vi "Actor Core.vi"(8 "error in":errorcluster, 11 "CANopen Test UI in":refnum<class "CANopen Test UI Actor.lvclass">) -> (0 "error out":errorcluster, 3 "Actor out":refnum<class "Actor.lvclass">)   [LabVIEW 2024, in "CANopen Test UI Actor.lvlib" / "CANopen Test UI Actor.lvclass"]
doc: "<p>(<strong>Filename</strong>: <span class=\"dnl\">Actor Framework.lvlib:Actor.lvclass:Actor Core.vi</span>)</p>\n<p>Receives messages to the actor, reacts to them, and initiates any error handling that may shut the actor down.</p>\n<p>Descendant classes may override this VI to append parallel tasks for the actor to complete while it handles messages. Overrides use the <a href=\"nihelplauncher://docs/csh?context=lvcore_glang_udclass\">Call Parent Class Method</a> node.</p>"
uses:
  CANopen Test UI Actor.lvclass
  CANopen Test UI Actor.lvclass/CANopen Test UI Actor.ctl
  CANopen Actor Interface/CANopen Actor Interface Messages/Enable Heartbeat Msg/Enable Heartbeat Msg.lvclass
  <vilib>/ActorFramework/Actor/Actor.lvclass
  CANopen Actor/CANopen Actor/CANopen Actor.lvclass
  <vilib>/ActorFramework/Stop Msg/Stop Msg.lvclass
  CANopen/CANopen.lvclass
  HAL/HAL/Devices/CAN Interfaces/PCAN/PCAN.lvclass
  HAL/HAL/Configurations/CFG Base/CFG Base.lvclass
  CANopen/Multiplexer.ctl
  DSP402/DriveMode.ctl
  DSP402/DSP402.lvclass
  DSP402/DriveState.ctl
  CANopen/Peer-To-Peer Function Code.ctl
panel:
  in  "Stop":bool
  in  "Tab Control":T1(tab)
  in  "NMT send":bool
  in  "Node ID (NMT)":u8=50 caption="Node ID"
  in  "Command specifier":u8(ring)=129 items=["Start remote node"=1, "Stop remote node"=2, "Enter pre-operational state"=128, "Reset node"=129, "Reset communication"=130]
  in  "SDO size":u8=2 caption="Bytes" format="%0d"
  in  "SDO read":bool
  in  "Multiplexor":T2={"Index"=4119, "Sub-Index"=0} {"Sub-Index" format="%.0x"; "Index" format="%.0x"}
  in  "SDO value":u32 caption="Value" format="%08x"
  in  "SDO write":bool
  in  "Node ID (SDO)":u8=50 caption="Node ID"
  in  "Remap TxPDO":bool
  in  "TxPDO map":cluster{"CobID":u32, "nBytes":u8}[](array[cluster])=[{"CobID"=434, "nBytes"=2}] {"CobID" format="%x"}
  out "Input image":bool[](array[boolean])
  in  "Remap RxPDO":bool
  in  "RxPDO map":cluster{"CobID":u32, "nBytes":u8}[](array[cluster])=[{"CobID"=562, "nBytes"=5}] {"CobID" format="%x"}
  in  "Output image":bool[](array[boolean])
  in  "Node ID (402)":u8 caption="Node ID"
  in  "State (402)":T3 caption="State"
  in  "Mode (402)":T4 caption="Mode" items=["Undefined"=0, "Profile Position Mode"=1, "Velocity Mode"=2, "Profile Velocity Mode"=3, "Torque Profile Mode"=4, "Homing Mode"=6, "Interpolated Position Mode"=7]
  in  "Position (402)":u32 caption="Position"
  in  "Speed (402)":i16=500 caption="Speed (RpM)"
  in  "Operation flags (402)":cluster{"ON":bool, "OFF":bool}[](array[cluster]) caption="Force bit 4, 5, 6 and Halt"
  in  "Acceleration (402)":u32=100 caption="Acc"
  in  "Deceleration (402)":u32=100 caption="Dec"
  in  "Get status (402)":bool
  in  "PDO unlink":bool
  in  "PDO link":bool
  in  "Node ID (link)":u8=50 caption="Node ID"
  in  "Function code (link)":T5={"EMCY"=1, "NMT Error Control"=14, "PDO1 (rx)"=4, "PDO1 (tx)"=3, "PDO2 (rx)"=6, "PDO2 (tx)"=5, "PDO3 (rx)"=8, "PDO3 (tx)"=7, "PDO4 (rx)"=10, "PDO4 (tx)"=9, "SDO (rx)"=12, "SDO (tx)"=11} caption="Function code"
  in  "Indices":cluster{"Communication":u32, "Mapping":u32}={"Communication"=6144, "Mapping"=6656} {"Mapping" format="%x"; "Communication" format="%x"}
  in  "Map":cluster{"Multiplexor":T2, "nBits":u8}[](array[cluster])=[{"Multiplexor"={"Index"=24832, "Sub-Index"=1}, "nBits"=16}] {"Multiplexor"."Sub-Index" format="%.0x"; "Multiplexor"."Index" format="%.0x"}
  in  "Heartbeat set":bool
  in  "Heartbeat table":T6(array[cluster]) {"Period" format="%#.3g"}
  in  "Raw send":bool
  in  "Data (raw)":u8[](array[numeric]) caption="Data" format="%02x"
  in  "Node ID (raw)":u8 caption="Node ID"
  in  "Function code (raw)":T5={"EMCY"=1, "NMT Error Control"=14, "PDO1 (rx)"=4, "PDO1 (tx)"=3, "PDO2 (rx)"=6, "PDO2 (tx)"=5, "PDO3 (rx)"=8, "PDO3 (tx)"=7, "PDO4 (rx)"=10, "PDO4 (tx)"=9, "SDO (rx)"=12, "SDO (tx)"=11}
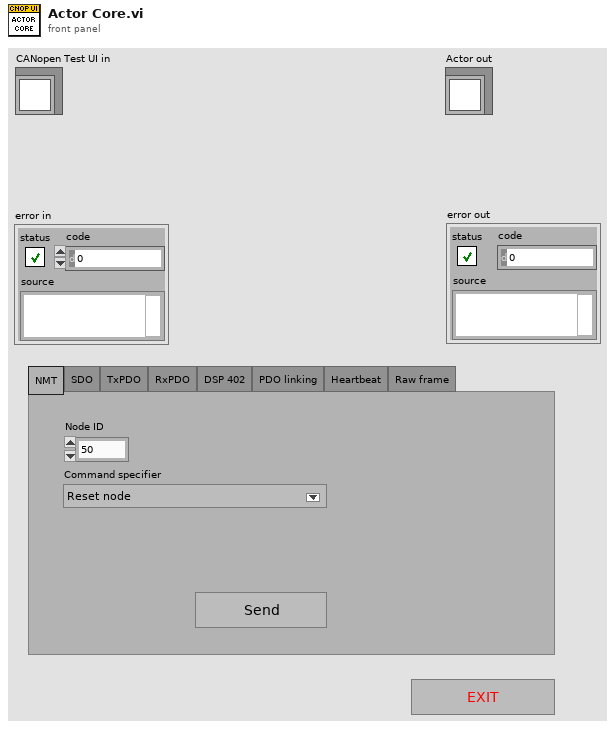
[diagram p1: front panel]
types:
  T1 = enum32{"NMT", "SDO", "TxPDO", "RxPDO", "DSP 402", "PDO linking", "Heartbeat", "Raw frame"}
  T2 = typedef "canopen.lvlib/CANopen.lvclass/Multiplexer.ctl" = cluster{"Index":u16, "Sub-Index":u8}
  T3 = typedef "canopen.lvlib/DSP402.lvclass/DriveState.ctl" = enum16{"Start", "Not ready to switch on", "Switch on disabled", "Ready to switch on", "Switched on", "Operation enable", "Fault reaction active", "Fault", "Quick stop active"}
  T4 = typedef "canopen.lvlib/DSP402.lvclass/DriveMode.ctl" = i8
  T5 = typedef "Peer-To-Peer Function Code.ctl" = map{string, i32}
  T6 = cluster{"Node ID":u8, "Period":dbl, "Set value":i16, "Value":i16}[]
  T7 = cluster{"Node ID":u8, "Period":dbl, "Set value":i16, "Value":i16}
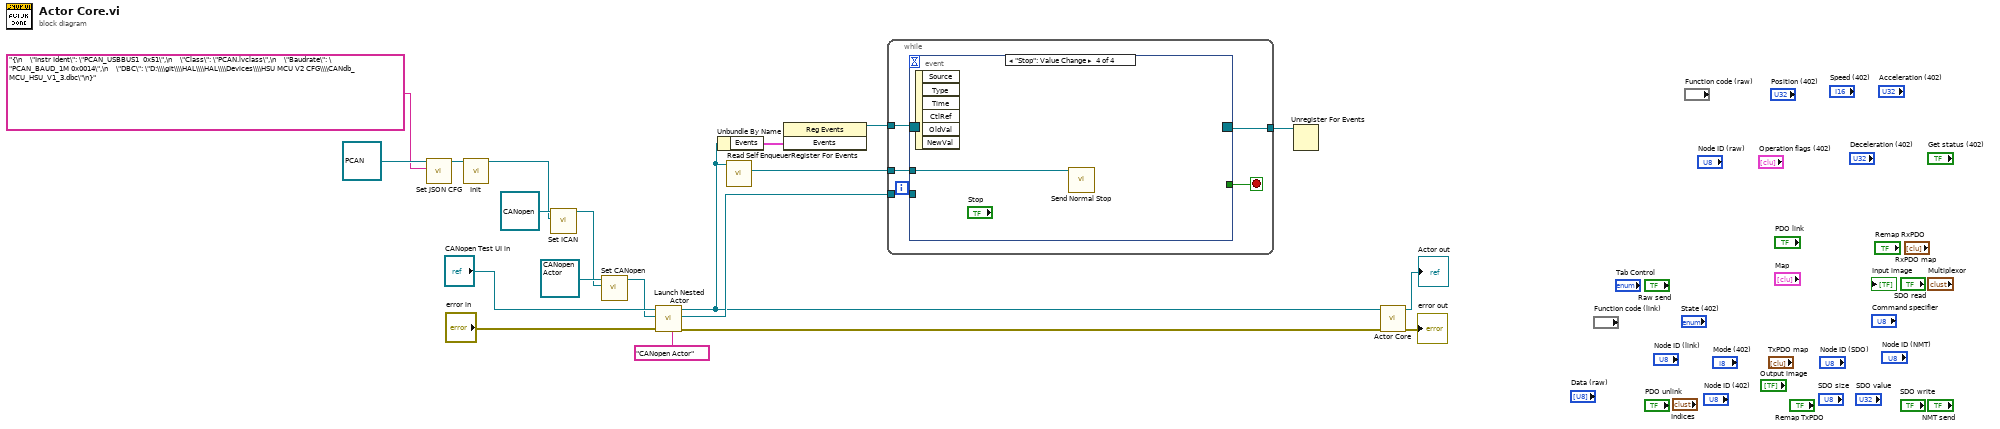
[diagram p0: block diagram]
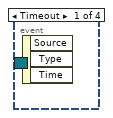
[diagram p2: hidden frame]
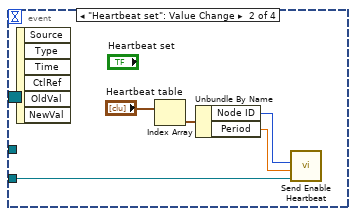
[diagram p3: hidden frame]
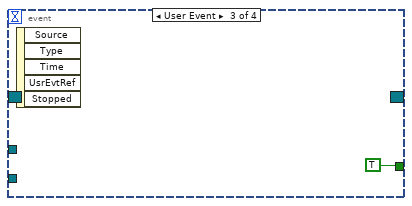
[diagram p4: hidden frame]
diagram:
  n1 = call "Set JSON CFG.vi"("<JSON>CFG"="{\n    \"Instr Ident\": \"PCAN_USBBUS1  0x51\",\n    \"Class\": \"PCAN.lvclass\",\n    \"Baudrate\": \"PCAN_BAUD_1M 0x0014\",\n    \"DBC\": \"D:\\\\git\\\\HAL\\\\HAL\\\\Devices\\\\HSU MCU V2 CFG\\\\CANdb_MCU_HSU_V1_3.dbc\"\n}", "CFG Base in"=refnum<class "PCAN.lvclass"> refnum ("PCAN.lvclass")) -> ("CFG Base out"=w3:refnum<class "PCAN.lvclass">)  [unwired: 9 in]
  n2 = call-dynamic "Init.vi"("PCAN in"=w3) -> ("PCAN out"=w1:refnum<class "PCAN.lvclass">)  [unwired: 9 in, 1 out]
  n3 = call "Set ICAN.vi"("ICAN"=w1, "CANopen in"=refnum<class "CANopen.lvclass"> refnum ("CANopen.lvlib:CANopen.lvclass")) -> ("CANopen out"=w5:refnum<class "CANopen.lvclass">)  [unwired: 9 in]
  n4 = call "Set CANopen.vi"("CANopen"=w5, "CANopen Actor in"=refnum<class "CANopen Actor.lvclass"> refnum ("CANopen Actor.lvlib:CANopen Actor.lvclass")) -> ("CANopen Actor out"=w8:refnum<class "CANopen Actor.lvclass">)  [unwired: 9 in]
  n5 = call <vilib>:"Launch Nested Actor.vi"("Debug Alias"="CANopen Actor", "error in (no error)"="error in", "Nested Actor"=w8, "Caller Actor in"="CANopen Test UI in") -> ("error out"=w16:errorcluster, "Nested Actor's Enqueuer"=w15:refnum<class "Message Enqueuer.lvclass">, "Caller Actor out"=w12:refnum<class "CANopen Test UI Actor.lvclass">)  [unwired: 5 in]
  n6 = Unbundle By Name(w12) -> ("Events"=w11:cluster{"Stopped":refnum<user-event>})
  n7 = call <vilib>:"Read Self Enqueuer.vi"("Actor"=w12) -> ("Self Enqueuer"=w13:refnum<class "Message Enqueuer.lvclass">)  [unwired: 10 in]
  n8 = register-events(w11) -> (reference out=w10:refnum<event-registration>)  [unwired: 2 in, 1 out]
  n9 = while {
    tunnel: [w25] -> w18
    tunnel: w15 -> [w24]
    tunnel: w13 -> [w23]
    tunnel: w10 -> [w22]
    stop <- w21 stop-if-true
    n10 = event shown="[3] \"Stop\": Value Change" {
      selector: w22 -> [_ _ _ _]
      dyn-events: [_ _ _ _] -> w25
      timeout: _ -> [_ _ _ _]
      tunnel: w24 -> [_ w26 _ _]
      tunnel: w23 -> [_ _ _ w32]
      tunnel: [_ _ TRUE _] -> w21
      event Timeout {
        n11 = event-data() -> ()  [unwired: 1 in, 3 out]
      }
      event "Heartbeat set": Value Change {
        n12 = event-data() -> ()  [unwired: 1 in, 6 out]
        n13 = Index Array(array="Heartbeat table") -> (element=w29:T7)  [unwired: 1 in]
        n14 = Unbundle By Name(w29) -> ("Node ID"=w27:u8, "Period"=w28:dbl)
        n15 = call "Send Enable Heartbeat.vi"("Period"=w28, "Node ID"=w27, "Message Enqueuer"=w26) -> ()  [unwired: 7 in, 2 out]
      }
      event User Event {
        n16 = event-data() -> ()  [unwired: 1 in, 5 out]
      }
      event "Stop": Value Change {
        n17 = event-data() -> ()  [unwired: 1 in, 6 out]
        n18 = call <vilib>:"Send Normal Stop.vi"("Message Enqueuer"=w32) -> ()  [unwired: 10 in, 1 out]
      }
    }
  }
  n19 = Unregister For Events(event registration refnum=w18) -> ()  [unwired: 1 in, 1 out]
  n20 = call-parent "Actor Core.vi"("error in"=w16, "Actor in"=w12) -> ("error out"=→"error out":errorcluster, "Actor out"=→"Actor out":refnum<class "Actor.lvclass">)  [unwired: 8 in]
